vi "Next Temperature Cycle.vi"(8 "error in (no error)":errorcluster, 11 "Temperature Control in":refnum<class "Temperature Control.lvclass">) -> (0 "error out":errorcluster, 1 "Set Point":T1, 2 "Temperature Finished":bool, 3 "Temperature Control out":refnum<class "Temperature Control.lvclass">)   [LabVIEW 2020, in "Temperature Control.lvclass"]
doc: "Steps to the next temperature cycle.\nIf no more cycles are defined it stops the cycle"
uses:
  Temperature Control.lvclass
  Controls/Set point.ctl
  Temperature Control.lvclass/Temperature Control.ctl
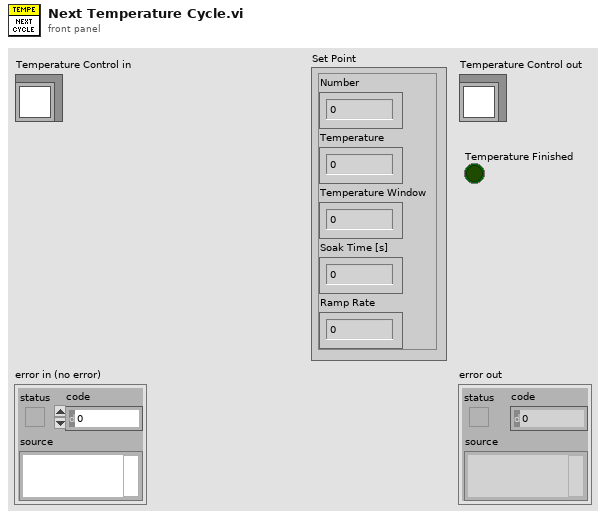
[diagram p1: front panel]
types:
  T1 = typedef "Temperature Control.lvclass/Set point.ctl" = cluster{"Number":u32, "Temperature":dbl, "Temperature Window":dbl, "Soak Time [s]":u32, "Ramp Rate":dbl}
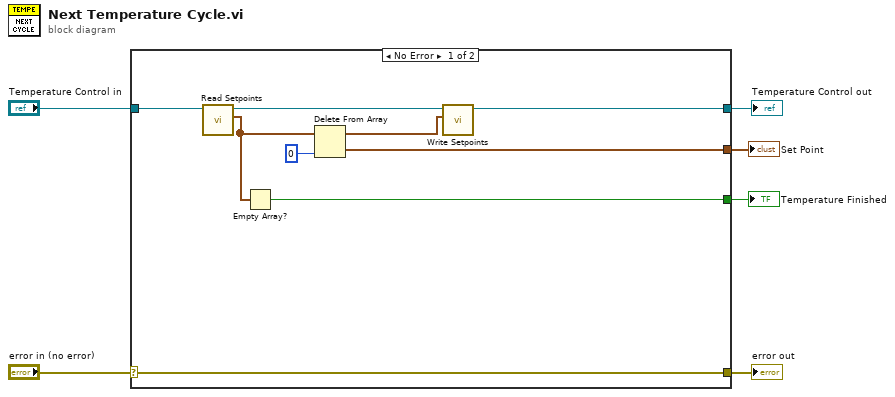
[diagram p0: block diagram]
diagram:
  n1 = case shown="No Error" "error in (no error)" {
    selector: "error in (no error)" -> [w15 w17]
    tunnel: [w15 w17] -> w5
    tunnel: [w9 w16] -> w3
    tunnel: "Temperature Control in" -> [w14 w16]
    tunnel: [w11 _] -> w2
    tunnel: [w7 _] -> w1
    frame No Error {
      n2 = call "Read Setpoints.vi"("Temperature Control in"=w14) -> ("Setpoints"=w13:T1[], "Temperature Control out"=w10:refnum<class "Temperature Control.lvclass">)  [unwired: 9 in]
      n3 = Empty Array?(array=w13) -> (empty?=w11:bool)
      n4 = Delete From Array(array=w13, index=0) -> (deleted portion=w7:T1, array with subset deleted=w8:T1[])  [unwired: 1 in]
      n5 = call "Write Setpoints.vi"("Setpoints"=w8, "Temperature Control in"=w10) -> ("Temperature Control out"=w9:refnum<class "Temperature Control.lvclass">)  [unwired: 9 in]
    }
    frame Error {
    }
  }
  "error out" <- w5
  "Temperature Control out" <- w3
  "Temperature Finished" <- w2
  "Set Point" <- w1
